vi "LoginForm.vi"() -> ()   [LabVIEW 2025]
uses:
  <vilib>/httpClient/POSTBuffer.vi
  <vilib>/httpClient/LabVIEWHTTPClient.lvlib
panel:
  in  "?":cluster{"email":string, "password":string}
  in  "?":bool
  # "Login"
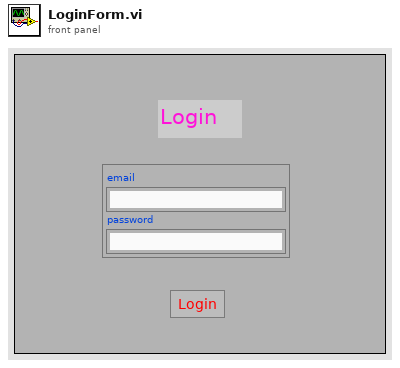
[diagram p1: front panel]
types:
  T1 = enum8{"Enabled", "Disabled", "Disabled and Grayed Out"}
  T2 = typedef "LabVIEWHTTPClient.lvlib/ClientHandle.ctl" = refnum<k1>
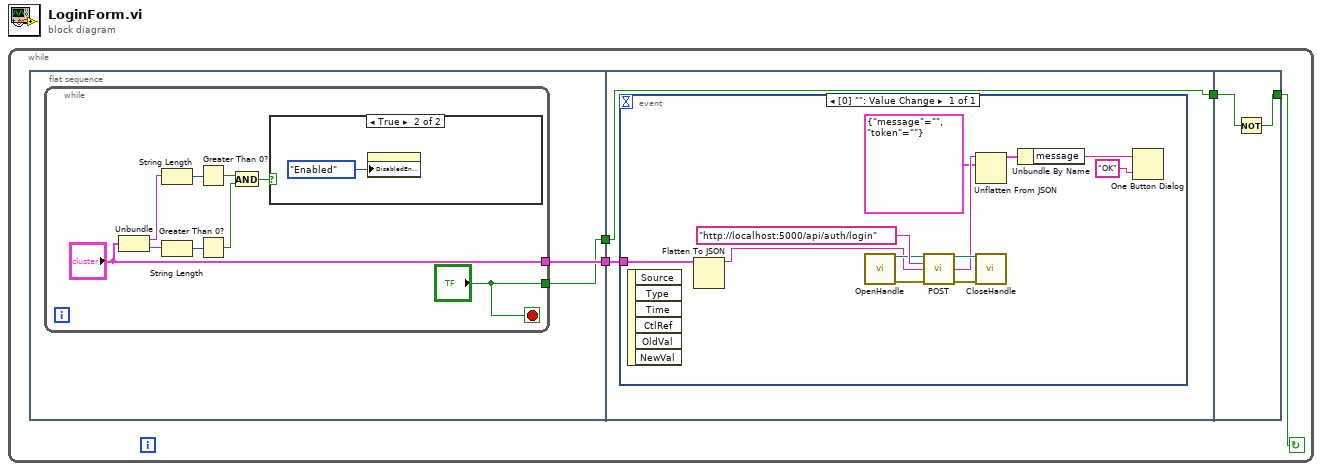
[diagram p0: block diagram]
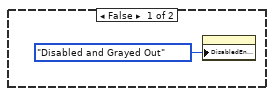
[diagram p2: hidden frame]
diagram:
  n1 = while {
    stop <- w4 continue-if-true
    n2 = flat-sequence {
      tunnel: [w5] -> w2
      tunnel: [w6] -> w1
      tunnel: [w19] -> w3
      tunnel: w2 -> [w19]
      tunnel: w1 -> [w18]
      tunnel: [w32] -> w4
      tunnel: w3 -> [w33]
      frame #0 {
        n3 = while {
          tunnel: ["?"] -> w6
          tunnel: ["?"] -> w5
          stop <- "?" stop-if-true
          n4 = Unbundle("?") -> ("email"=w10:string, "password"=w9:string)
          n5 = String Length(string=w10) -> (length=w14:i32)
          n6 = String Length(string=w9) -> (length=w13:i32)
          n7 = Greater Than 0?(x=w14) -> (x > 0?=w15:bool)
          n8 = Greater Than 0?(x=w13) -> (x > 0?=w12:bool)
          n9 = And(x=w15, y=w12) -> (x .and. y?=w11:bool)
          n10 = case shown="True" w11 {
            frame False {
              n11 = property class="Bool"("DisabledEnum"=T1."Disabled and Grayed Out" ("Disabled")) -> ()  [unwired: 2 in, 2 out]
            }
            frame True {
              n12 = property class="Bool"("DisabledEnum"=T1."Enabled" ("Disabled")) -> ()  [unwired: 2 in, 2 out]
            }
          }
        }
      }
      frame #1 {
        n13 = event shown="[0] \"\": Value Change" {
          selector: _ -> [_]
          dyn-events: _ -> [_]
          timeout: _ -> [_]
          tunnel: w18 -> [w21]
          event Value Change {
            n14 = event-data() -> ()  [unwired: 1 in, 6 out]
            n15 = Flatten To JSON(anything=w21) -> (JSON string=w26:string)  [unwired: 2 in, 1 out]
            n16 = call <vilib>:"OpenHandle.vi"() -> ("client handle out"=w29:T2, "error out"=w30:errorcluster)  [unwired: 14 in]
            n17 = call-poly <vilib>:"POST.vi"("client handle"=w29, "url"="http://localhost:5000/api/auth/login", "buffer"=w26, "error in (no error)"=w30) -> ("client handle out"=w28:T2, "body"=w24:string, "error out"=w27:errorcluster)  [unwired: 8 in, 1 out]
            n18 = Unflatten From JSON(JSON string=w24, type and defaults=cluster{"message":string, "token":string} {"message"="", "token"=""}) -> (value=w23:cluster{"message":string, "token":string})  [unwired: 5 in, 1 out]
            n19 = call <vilib>:"CloseHandle.vi"("client handle"=w28, "error in (no error)"=w27) -> ()  [unwired: 13 in, 1 out]
            n20 = Unbundle By Name(w23) -> ("message"=w22:string)
            n21 = One Button Dialog(message=w22, button name ("OK")="OK") -> ()  [unwired: 1 out]
          }
        }
      }
      frame #2 {
        n22 = Not(x=w33) -> (.not. x?=w32:bool)
      }
    }
  }
